vi "NI VeriStand - Start Waveform(s).vi"   [LabVIEW 2020, in "NI_VS Custom Device Waveform API.lvlib"]
doc: "Sets the start time (t0) for the waveform data you want to write with the Write Waveform(s) VI. NI VeriStand considers all data the custom device writes to a waveform be continuous unless this VI executes again with a different start time."
uses:
  <vilib>/NI VeriStand/Custom Device Waveform API/NI_VS Custom Device Waveform API.lvlib
  <vilib>/NI VeriStand/Custom Device Waveform API/Single Waveform Write (DBL)/Single Waveform Write (DBL).lvclass
  <vilib>/NI VeriStand/Custom Device Waveform API/Multiple Waveforms Write (DBL)/Multiple Waveforms Write (DBL).lvclass
  <vilib>/NI VeriStand/Custom Device Waveform API/Single Waveform Write (CDB)/Single Waveform Write (CDB).lvclass
  <vilib>/NI VeriStand/Custom Device Waveform API/Multiple Waveforms Write (CDB)/Multiple Waveforms Write (CDB).lvclass
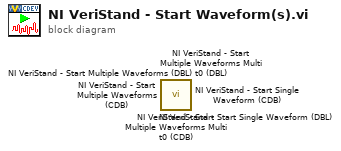
[diagram p0: block diagram]
diagram:
  n1 = call <vilib>:"NI VeriStand - Start Multiple Waveforms Multi t0 (CDB).vi"() -> ()  [unwired: 10 in, 2 out]
  n2 = call <vilib>:"NI VeriStand - Start Multiple Waveforms Multi t0 (DBL).vi"() -> ()  [unwired: 10 in, 2 out]
  n3 = call <vilib>:"NI VeriStand - Start Multiple Waveforms (CDB).vi"() -> ()  [unwired: 10 in, 2 out]
  n4 = call <vilib>:"NI VeriStand - Start Single Waveform (CDB).vi"() -> ()  [unwired: 10 in, 2 out]
  n5 = call <vilib>:"NI VeriStand - Start Multiple Waveforms (DBL).vi"() -> ()  [unwired: 10 in, 2 out]
  n6 = call <vilib>:"NI VeriStand - Start Single Waveform (DBL).vi"() -> ()  [unwired: 10 in, 2 out]
